vi "Tegam4040 - DAC.vi"(0 "Instrument Session Handle In":u32 format="%x", 7 "DAC":u32 max=65535 format="%x", 11 "error in (no error)":errorcluster) -> (4 "Instrument Session Handle Out (dupl)":u32 format="%x", 15 "error out":errorcluster)   [LabVIEW 2010, in "Tegam4040.lvlib"]
doc: "DAC Control:\n\nMust use INIT VI to get DAC in know state of 7FFF. This VI will not read back DAC value as other VI's it will set the Value only."
uses:
  Tegam4040.lvlib
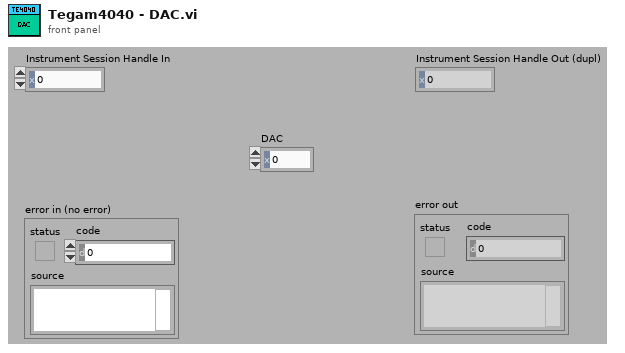
[diagram p1: front panel]
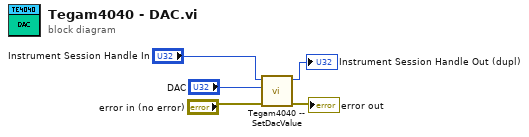
[diagram p0: block diagram]
diagram:
  n1 = call "Tegam4040 -- SetDacValue.vi"("error in (no error)"="error in (no error)", "DAC Value"="DAC", "Instrument Session Handle In"="Instrument Session Handle In") -> ("error out"=→"error out":errorcluster, "Instrument Session Handle Out (dupl)"=→"Instrument Session Handle Out (dupl)":u32)  [unwired: 7 in]
